vi "Pre Launch Init.vi"(11 "Caller in":refnum<class "Caller.lvclass">) -> (0 "error out":errorcluster, 3 "Caller out":refnum<class "Caller.lvclass">)   [LabVIEW 2020, in "Caller.lvlib" / "Caller.lvclass"]
doc: "(<B>Filename</B>: Actor Framework.lvlib:Actor.lvclass:Pre Launch Init.vi)\n\nDefines behavior that occurs after the Launch Nested Actor method is invoked but before the actor's Actor Core method begins running.\n\nBy default, this method does nothing. A descendant class may override it to define behavior."
uses:
  Caller.lvclass
  C:/Program Files/National Instruments/LabVIEW 2020/vi.lib/ActorFramework/Actor/Actor.lvclass
  Caller.lvclass/Caller.ctl
  <vilib>/ActorFramework/Actor/Actor.lvclass/Actor.ctl
  <vilib>/ActorFramework/Message Enqueuer/Message Enqueuer.lvclass/Message Enqueuer.ctl
  <vilib>/ActorFramework/Message Enqueuer/Init from Existing Queue.vi
  <vilib>/ActorFramework/Actor/Actor.lvclass
  <vilib>/ActorFramework/Message Enqueuer/Message Enqueuer.lvclass
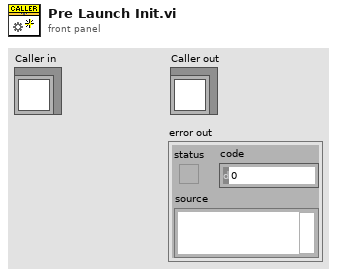
[diagram p1: front panel]
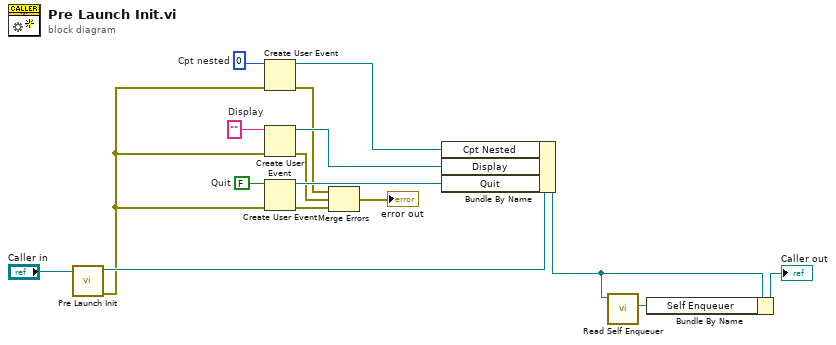
[diagram p0: block diagram]
diagram:
  w2 = u8 0  # Cpt nested
  w8 = ""  # Display
  w16 = FALSE  # Quit
  n1 = call-parent "Pre Launch Init.vi"("Actor in"="Caller in") -> ("error out"=w4:errorcluster, "Actor out"=w11:refnum<class "Caller.lvclass">)  [unwired: 9 in]
  n2 = Create User Event(user event datatype=w2, error in=w4) -> (user event=w1:refnum<user-event>, error out=w3:errorcluster)
  n3 = Create User Event(user event datatype=w8, error in=w4) -> (user event=w5:refnum<user-event>, error out=w6:errorcluster)
  n4 = Create User Event(user event datatype=w16, error in=w4) -> (user event=w15:refnum<user-event>, error out=w9:errorcluster)
  n5 = Merge Errors(w3, w6, w9) -> (→"error out":errorcluster)
  n6 = Bundle By Name(cluster=w11, "Cpt Nested"=w1, "Display"=w5, "Quit"=w15) -> (w10:refnum<class "Caller.lvclass">)
  n7 = call <vilib>:"Read Self Enqueuer.vi"("Actor"=w10) -> ("Self Enqueuer"=w13:refnum<class "Message Enqueuer.lvclass">)  [unwired: 10 in]
  n8 = Bundle By Name(cluster=w10, "Self Enqueuer"=w13) -> (→"Caller out":refnum<class "Caller.lvclass">)
